vi "Deserialize Pixel Data.vi"(9 "Input Valid":bool, 10 "Ready For Output":bool, 11 "Pixel Data":bool[](array[boolean])=[FALSE, FALSE, FALSE, FALSE, FALSE, FALSE, FALSE, FALSE]) -> (1 "Ready For Input":bool, 2 "Output Valid":bool, 3 "Deserialized Data":bool)   [LabVIEW 2021, in "Neopixel - FPGA.lvclass"]
uses:
  Neopixel - FPGA.lvclass
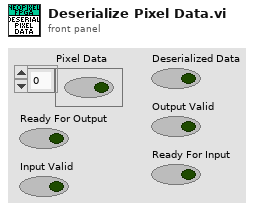
[diagram p1: front panel]
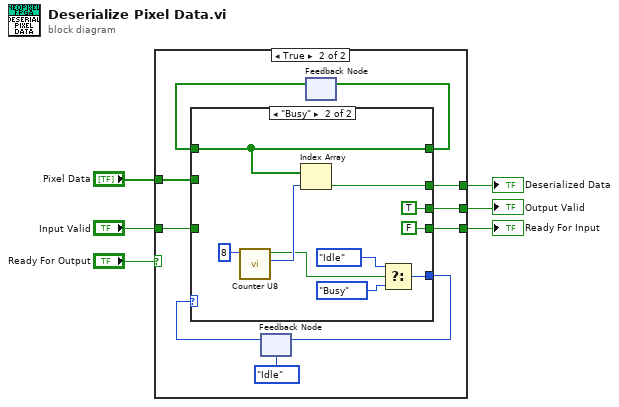
[diagram p0: block diagram]
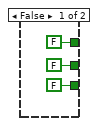
[diagram p2: hidden frame]
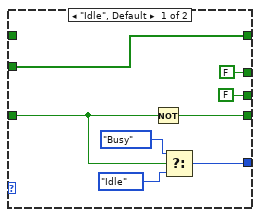
[diagram p3: hidden frame]
diagram:
  n1 = case shown="True" "Ready For Output" {
    tunnel: "Pixel Data" -> [_ w19]
    tunnel: "Input Valid" -> [_ w16]
    tunnel: [FALSE ("Value Reached") w15] -> w4
    tunnel: [FALSE w11] -> w3
    tunnel: [FALSE w10] -> w2
    frame False {
    }
    frame True {
      n2 = feedback #1(enum8{"Idle", "Busy"}."Idle") -> (w17:enum8{"Idle", "Busy"})
      n3 = feedback #2() -> (w13:bool[])  [unwired: 1 in]
      n4 = case shown="\"Busy\"" w17 {
        tunnel: w19 -> [w22 _]
        tunnel: w16 -> [w27 _]
        tunnel: [w26 FALSE] -> w15
        tunnel: [w23 w30] -> w14
        tunnel: w13 -> [_ w35]
        tunnel: [w22 w35] -> w12
        tunnel: [FALSE w36] -> w11
        tunnel: [FALSE TRUE] -> w10
        frame "Idle", Default {
          n5 = Not(x=w27) -> (.not. x?=w26:bool)
          n6 = Select(t=enum8{"Idle", "Busy"}."Busy", s=w27, f=enum8{"Idle", "Busy"}."Idle") -> (s? t:f=w23:enum8{"Idle", "Busy"})
        }
        frame "Busy" {
          n7 = call "Counter U8.vi"("Count To"=u8 8) -> ("Current Value"=w33:u8, "Value Reached"=w29:bool)  [unwired: 9 in]
          n8 = Index Array(array=w35, index=w33) -> (element=w36:bool)
          n9 = Select(t=enum8{"Idle", "Busy"}."Idle", s=w29, f=enum8{"Idle", "Busy"}."Busy") -> (s? t:f=w30:enum8{"Idle", "Busy"})
        }
      }
      n10 = feedback-in #1(w14) -> ()
      n11 = feedback-in #2(w12) -> ()
    }
  }
  "Deserialized Data" <- w3
  "Ready For Input" <- w4
  "Output Valid" <- w2
